vi "Check If Date Is Fit.vi"(8 "error in (no error)":errorcluster, 9 "CurWeek(0)":i32, 10 "Path":path, 11 "CalAttendance in":refnum<class "CalAttendance.lvclass">) -> (0 "error out":errorcluster, 2 "Fit(False)":bool, 3 "CalAttendance out":refnum<class "CalAttendance.lvclass">)   [LabVIEW 2015, in "Admin_Actor.lvlib" / "CalAttendance.lvclass"]
uses:
  CalAttendance.lvclass
  Models/ExcelReader/ExcelReader.lvclass
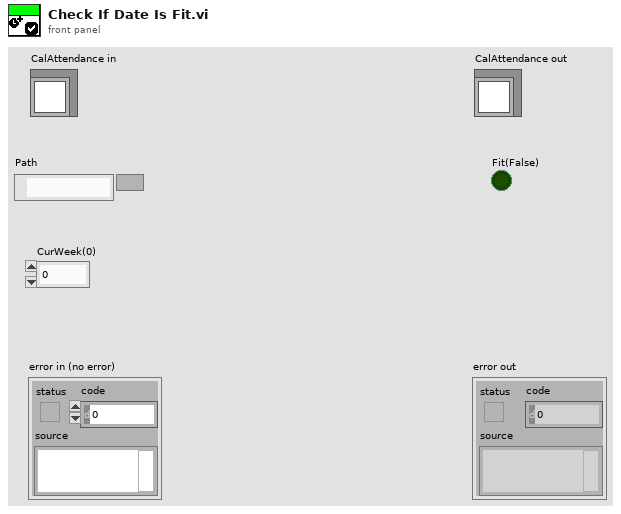
[diagram p1: front panel]
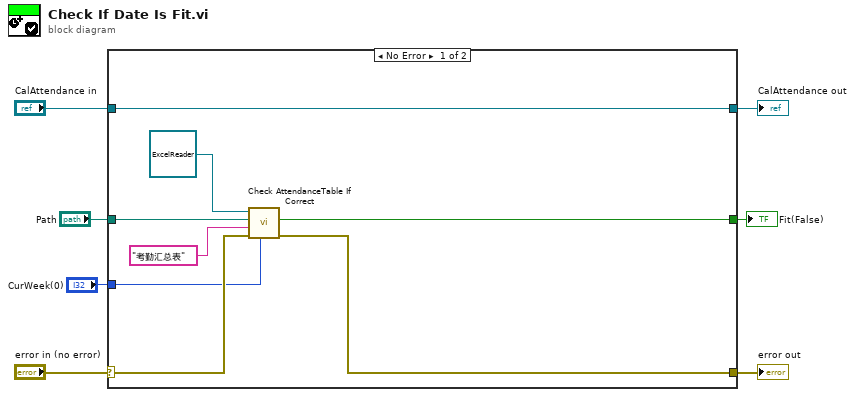
[diagram p0: block diagram]
diagram:
  n1 = case shown="No Error" "error in (no error)" {
    selector: "error in (no error)" -> [w13 w17]
    tunnel: [w9 w17] -> w6
    tunnel: [w15 w16] -> w4
    tunnel: "CalAttendance in" -> [w15 w16]
    tunnel: "Path" -> [w12 _]
    tunnel: "CurWeek(0)" -> [w10 _]
    tunnel: [w8 _] -> w1
    frame No Error {
      n2 = call "Check AttendanceTable If Correct.vi"("CurWeek(0)"=w10, "error in (no error)"=w13, "SheetName(\"\")"="考勤汇总表" ("SheetName(\"\")"), "Path"=w12, "ExcelReader in"=refnum<class "ExcelReader.lvclass"> refnum) -> ("error out"=w9:errorcluster, "Fit(False)"=w8:bool)  [unwired: 4 in, 1 out]
    }
    frame Error {
    }
  }
  "error out" <- w6
  "CalAttendance out" <- w4
  "Fit(False)" <- w1
